vi "FR Measure.vi"(6 "AC sync source":T1, 8 "FR measurement":T6={"Measurement frequencies (Hz)"=[1000.0, 10000.0, 1000.0], "Sampling frequency (Hz)"=500000.0, "Signal amplitude (V)"=4.5, "AC-DC settle time (s)"=20.0, "Record length (multiples of period)"=[1000.0, 10000.0, 1000.0], "Measurement template file"=path "", "Row of START keyword"=0, "Row of STOP keyword"=0, "Calculate RMS from samples"=FALSE, "AC-DC warm up time (s)"=300.0, "Measurement template line"=[], "DC meter readings No."=10, "Algorithm"="TWM-WFFT", "Simultaneous measurement"=FALSE, "Recalculate-skip already calculated"=FALSE} {"Record length (multiples of period)" format="%#_3p"; "Sampling frequency (Hz)" format="%#_3p"; "Measurement frequencies (Hz)" format="%#_3p"}, 9 "DC meter":T4={"DC meter type"=enum."H/A/K 3458", "DC meter VISA"="", "NPLC"=10.0, "status ref"=refnum}, 10 "AC Source":T1, 11 "Common properties":T3={"Measurement status ref"=refnum, "TWM Status ref"=refnum, "Abort ref"=refnum, "Skip waiting ref"=refnum, "GNU Octave path"=path "C:/Program Files/GNU Octave/Octave-6.2.0/mingw64/bin", "TWM+QWTB path"=path "C:/Users/labina/Desktop/TWM-1.8.7.0-full/octprog", "lvlib path"=path "D:/martin/WAC/WACsw - github/control_software/Filter function meter/external libraries/GOLPI 0.7.3.1 source distribution LV 20.0 32 bit/lv_proc.dll", "TWM pipe"="\\\\.\\pipe\\TWM:server", "PJVS status ref"=refnum, "WAC path"=path ""}) -> (0 "error out":errorcluster)   [LabVIEW 2020]
doc: "Main VI to run digitizer frequency response. Setup devices, run loop for all freuencies, stop devices."
uses:
  Type definitions/FR measuement.ctl
  General DC meter/Type definitions/DC meter.ctl
  General DC meter/Type definitions/DC meter type.ctl
  General AC source/Type definitions/AC Source.ctl
  General AC source/Type definitions/AC Source type.ctl
  Utilities/Type definitions/Common properties.ctl
  <vilib>/Utility/error.llb/DialogType.ctl
  <vilib>/Utility/NIReport.llb/NI_report.lvclass
  external libraries/varilib/varilib.lvlib
  external libraries/TWM-1.8.7.0-client/TWM Client.lvlib
panel:
  out "TWM handle":i32
  out "DC readings of AC-AC sequence":dbl[][](array[numeric])
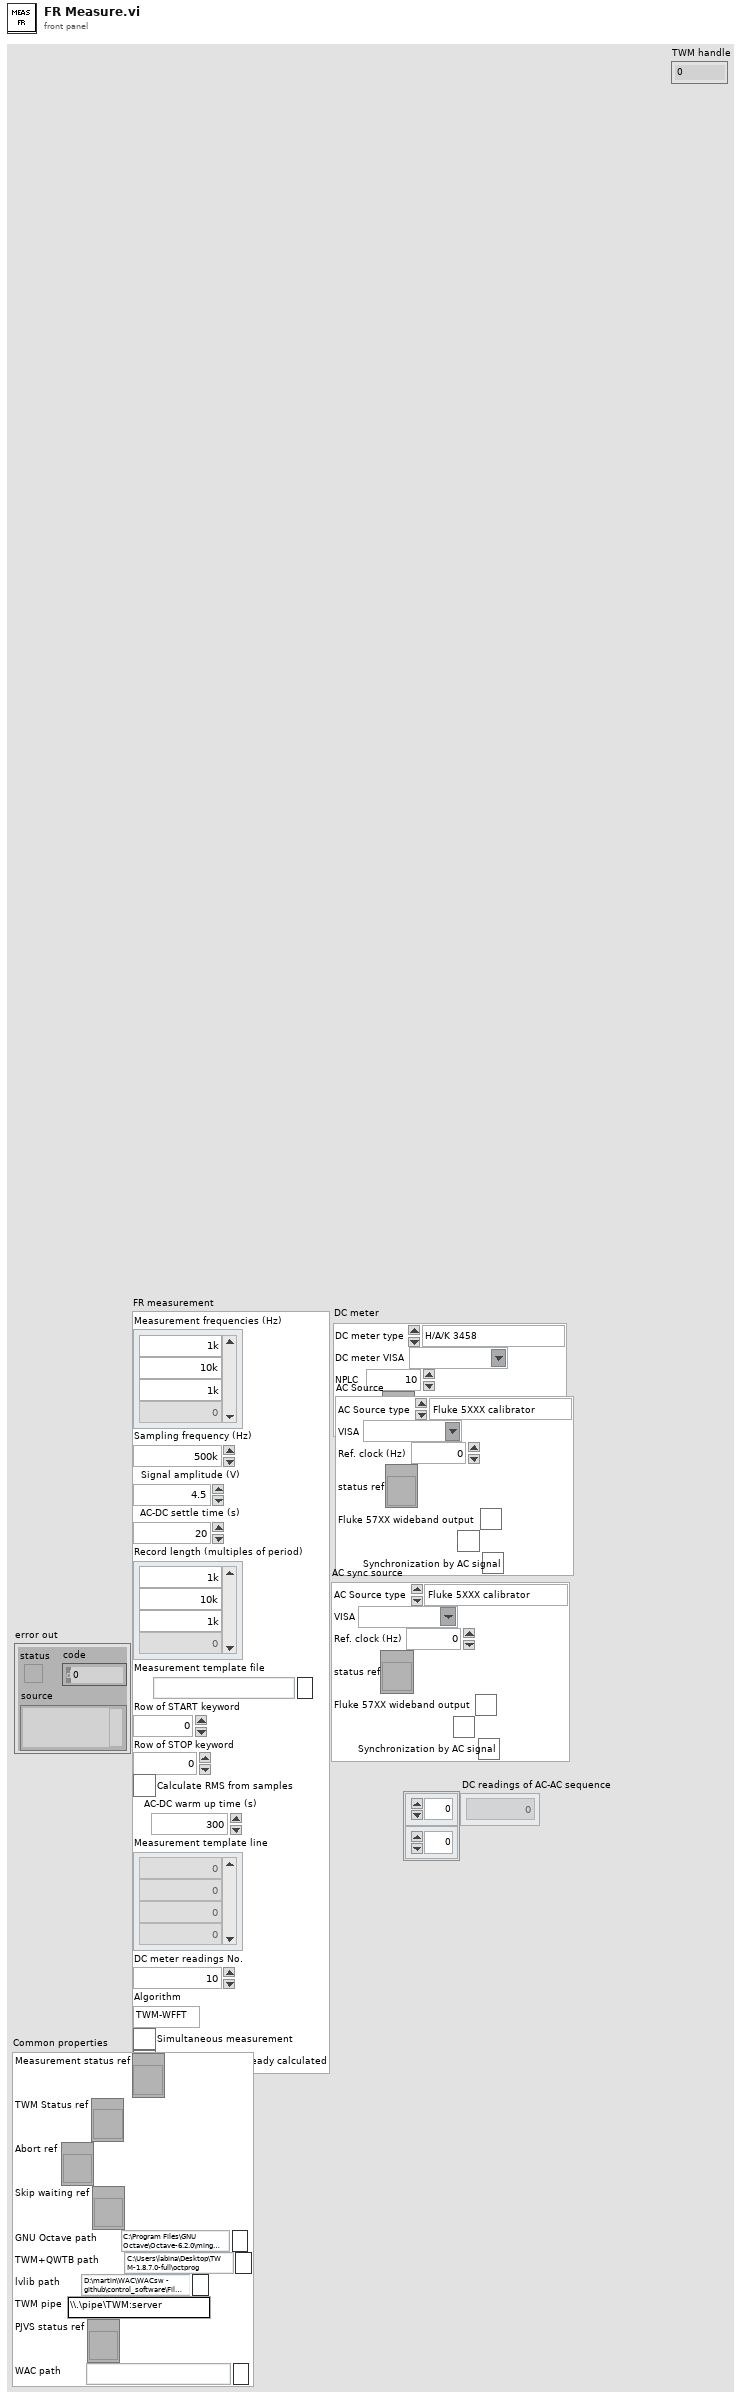
[diagram p1: front panel]
types:
  T1 = typedef "AC Source.ctl" = cluster{"AC Source type":T2, "VISA":refnum<visa-resource-name>, "Ref. clock (Hz)":dbl, "status ref":refnum<vi>, "Fluke 57XX wideband output":bool, "Fluke 57XX ignore errors":bool, "Synchronization by AC signal":bool}
  T2 = typedef "AC Source type.ctl" = enum16{"Fluke 5XXX calibrator", "Tektronix AFG3000 series", "dummy", "Agilent 331xxA to 332xxA", "Agilent 335xxA to 336xxA"}
  T3 = typedef "Common properties.ctl" = cluster{"Measurement status ref":refnum<vi>, "TWM Status ref":refnum<vi>, "Abort ref":refnum<vi>, "Skip waiting ref":refnum<vi>, "GNU Octave path":path, "TWM+QWTB path":path, "lvlib path":path, "TWM pipe":string, "PJVS status ref":refnum<vi>, "WAC path":path}
  T4 = typedef "DC meter.ctl" = cluster{"DC meter type":T5, "DC meter VISA":refnum<visa-resource-name>, "NPLC":dbl, "status ref":refnum<vi>}
  T5 = typedef "DC meter type.ctl" = enum16{"H/A/K 3458", "Fluke 8508A", "dummy", "Keithley 2182"}
  T6 = typedef "FR measuement.ctl" = cluster{"Measurement frequencies (Hz)":dbl[], "Sampling frequency (Hz)":dbl, "Signal amplitude (V)":dbl, "AC-DC settle time (s)":dbl, "Record length (multiples of period)":dbl[], "Measurement template file":path, "Row of START keyword":i32, "Row of STOP keyword":i32, "Calculate RMS from samples":bool, "AC-DC warm up time (s)":dbl, "Measurement template line":i32[], "DC meter readings No.":i32, "Algorithm":string, "Simultaneous measurement":bool, "Recalculate-skip already calculated":bool}
  T7 = typedef "DialogType.ctl" = u16
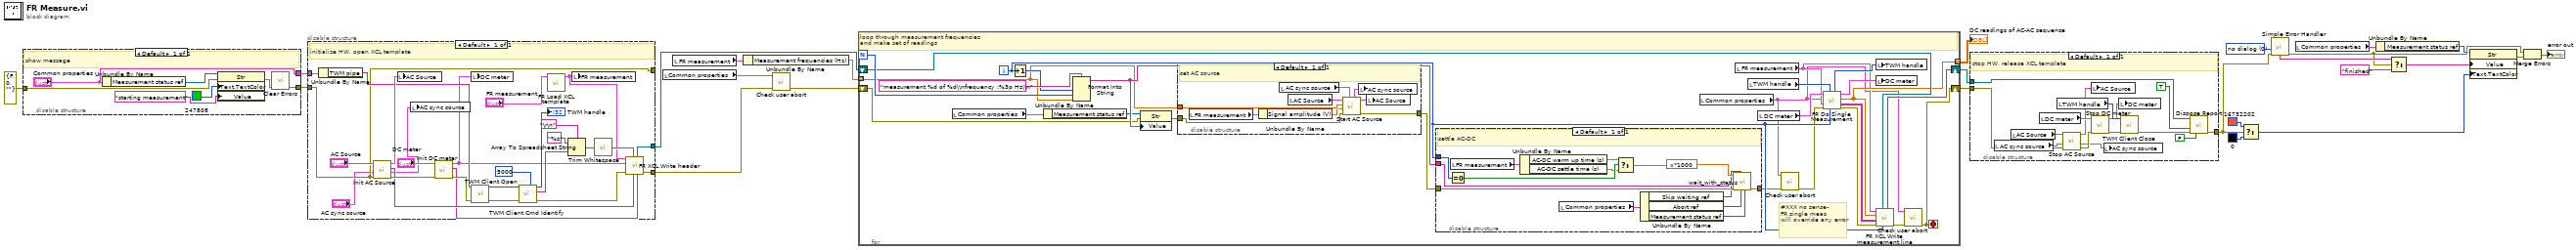
[diagram p0: block diagram]
diagram:
  w21 = T7 0 items=["no dialog", "OK message", "continue or stop message", "OK message + warnings", "continue/stop + warnings"] ("type of dialog (OK msg:1)")
  n1 = disable-structure shown="Default" {
    disable-tunnel: errorcluster {"status"=FALSE, "code"=0, "source"=""} ("error out") -> [w30]
    disable-tunnel: ["Common properties"] -> w2
    disable-tunnel: [w26] -> w1
    frame Enabled {
      # "show message"
      n2 = Unbundle By Name("Common properties") -> ("Measurement status ref"=w27:refnum<vi>)
      n3 = property class="Str"(reference=w27, error in=w30, "Text.TextColor"=u32 247808 ("Text.Text Colors:Text Color"), "Value"="starting measurement") -> (error out=w31:errorcluster)  [unwired: 1 out]
      n4 = call <vilib>:"Clear Errors.vi"("error in (no error)"=w31) -> ("error out"=w26:errorcluster)  [unwired: 5 in, 1 out]
    }
  }
  n5 = disable-structure shown="Default" {
    disable-tunnel: [w35] -> _
    disable-tunnel: [w57] -> w5
    disable-tunnel: [w56] -> w11
    disable-tunnel: w2 -> [w36]
    disable-tunnel: w1 -> [w35]
    frame Enabled {
      # "initialize HW, open XCL template"
      n6 = Unbundle By Name(w36) -> ("TWM pipe"=w40:string)
      n7 = call "Init AC Source.vi"("error in (no error)"=w35, "AC sync source"="AC sync source", "AC source"="AC Source") -> ("error out"=w59:errorcluster, "AC sync source out"=w33:T1, "Init status"=w55:string, "AC source out"=w42:T1)  [unwired: 5 in]
      n8 = local write "AC Source"(w42) -> ()
      n9 = local write "AC sync source"(w33) -> ()
      n10 = call "Init DC meter.vi"("error in (no error)"=w59, "DC meter"="DC meter") -> ("error out"=w58:errorcluster, "Init status"=w54:string, "DC meter out"=w39:T4)  [unwired: 7 in]
      n11 = local write "DC meter"(w39) -> ()
      n12 = call "TWM Client Open.vi"("error in"=w58, "pipe name"=w40) -> ("error out"=w49:errorcluster, "handle out"=w50:i32)  [unwired: 8 in]
      n13 = call "TWM Client Cmd Identify.vi"("timeout [ms]"=5000, "error in"=w49, "handle"=w50) -> ("error out"=w48:errorcluster, "channel idns"=w53:string[], "handle out"=→"TWM handle":i32)  [unwired: 5 in, 1 out]
      n14 = call "FR Load XCL template.vi"("FR measurement"="FR measurement") -> ("FR measurement out"=w37:T6)  [unwired: 10 in]
      n15 = Array To Spreadsheet String(delimiter (Tab)="\r\n", array=w53, 3:"%s" ("format string")) -> (spreadsheet string=w46:string)
      n16 = local write "FR measurement"(w37) -> ()
      n17 = call <vilib>:"Trim Whitespace.vi"("string"=w46) -> ("trimmed string"=w45:string)  [unwired: 1 in]
      n18 = call "FR XCL Write header.vi"("DC meter idn"=w54, "AC source idn"=w55, "Digitizer idn"=w45, "error in (no error)"=w48, "DC meter"=w39, "FR measurement"=w37) -> ("error out"=w57:errorcluster, "NI_report out"=w56:refnum<class "NI_report.lvclass">)  [unwired: 4 in]
    }
  }
  n19 = local read "Common properties"() -> (w3:T3)
  n20 = local read "FR measurement"() -> (w8:T6)
  n21 = Unbundle By Name(w8) -> ("Measurement frequencies (Hz)"=w7:dbl[])
  n22 = call "Check user abort.vi"("error in (no error)"=w5, "Common properties"=w3) -> ("error out"=w4:errorcluster)  [unwired: 9 in]
  n23 = for {
    N -> [w82]
    shift-right: [w66] -> w13
    shift-left: w4 -> [w78]
    tunnel: w7 -> [w79] mode=indexing
    tunnel: [w74] -> w25 mode=indexing
    shift-right: [w76] -> w10
    shift-left: w11 -> [w75]
    i -> [w73]
    stop <- w66 stop-if-true
    # "#XXX no sense-\nFR single meas \nwill override any error"
    # "loop through measurement frequencies\nand make set of readings"
    n24 = local read "Common properties"() -> (w71:T3)
    n25 = Increment(x=w73) -> (x+1=w83:i32)
    n26 = Unbundle By Name(w71) -> ("Measurement status ref"=w70:refnum<vi>)
    n27 = Format Into String(format string="measurement %d of %d\\nfrequency :%3p Hz\\n", w83, w82, w79) -> (resulting string=w84:string)  [unwired: 2 in, 1 out]
    n28 = property class="Str"(reference=w70, error in=w78, "Value"=w84) -> (error out=w81:errorcluster)  [unwired: 1 out]
    n29 = disable-structure shown="Default" {
      disable-tunnel: w81 -> [w108]
      disable-tunnel: [w107] -> w80
      disable-tunnel: w79 -> [w106]
      frame Enabled {
        # "set AC source"
        n30 = local read "FR measurement"() -> (w105:T6)
        n31 = Unbundle By Name(w105) -> ("Signal amplitude (V)"=w104:dbl)
        n32 = local read "AC sync source"() -> (w101:T1)
        n33 = local read "AC Source"() -> (w103:T1)
        n34 = call "Start AC Source.vi"("AC sync source"=w101, "error in (no error)"=w108, "Signal amplitude (V)"=w104, "Signal frequency  (Hz)"=w106, "AC source"=w103) -> ("error out"=w107:errorcluster, "AC source out"=w102:T1, "AC sync source out"=w100:T1)  [unwired: 3 in, 1 out]
        n35 = local write "AC sync source"(w100) -> ()
        n36 = local write "AC Source"(w102) -> ()
      }
    }
    n37 = disable-structure shown="Default" {
      disable-tunnel: w84 -> [w99]
      disable-tunnel: [w96] -> w62
      disable-tunnel: w80 -> [w98]
      disable-tunnel: w73 -> [w95]
      frame Enabled {
        # "settle AC-DC"
        n38 = Equal To 0?(x=w95) -> (x = 0?=w94:bool)
        n39 = local read "FR measurement"() -> (w88:T6)
        n40 = Unbundle By Name(w88) -> ("AC-DC warm up time (s)"=w87:dbl, "AC-DC settle time (s)"=w86:dbl)
        n41 = local read "Common properties"() -> (w92:T3)
        n42 = Select(t=w87, s=w94, f=w86) -> (s? t:f=w93:dbl)
        n43 = Unbundle By Name(w92) -> ("Skip waiting ref"=w91:refnum<vi>, "Abort ref"=w90:refnum<vi>, "Measurement status ref"=w89:refnum<vi>)
        n44 = expression code="x*1000"(w93) -> (w97:dbl)
        n45 = call "wait_with_status.vi"("stat ref"=w89, "stop ref"=w90, "second stop ref"=w91, "error in"=w98, "comment"=w99, "ms to wait"=w97) -> ("error out"=w96:errorcluster)  [unwired: 4 in, 1 out]
      }
    }
    n46 = local read "Common properties"() -> (w60:T3)
    n47 = local read "FR measurement"() -> (w63:T6)
    n48 = local read "TWM handle"() -> (w69:i32)
    n49 = local read "DC meter"() -> (w65:T4)
    n50 = call "Check user abort.vi"("error in (no error)"=w62, "Common properties"=w60) -> ("error out"=w61:errorcluster)  [unwired: 9 in]
    n51 = call "FR Do Single Measurement.vi"("Iteration index"=w73, "TWM handle in"=w69, "error in (no error)"=w61, "FR measurement"=w63, "Common properties"=w60, "DC meter"=w65) -> ("error out"=w77:errorcluster, "TWM result as string"=w72:string[][], "DC readings"=w74:dbl[], "DC meter out"=w64:T4, "TWM handle out"=w68:i32)  [unwired: 1 in]
    n52 = local write "TWM handle"(w68) -> ()
    n53 = local write "DC meter"(w64) -> ()
    n54 = call "FR XCL Write measurement line.vi"("Iteration index"=w73, "report in"=w75, "error in (no error)"=w77, "TWM result as string for XCL"=w72, "DC readings"=w74, "FR measurement"=w63) -> ("error out"=w67:errorcluster, "report out"=w76:refnum<class "NI_report.lvclass">)  [unwired: 4 in]
    n55 = call "Check user abort.vi"("error in (no error)"=w67, "Common properties"=w60) -> ("error out"=w66:errorcluster)  [unwired: 9 in]
  }
  "DC readings of AC-AC sequence" <- w25
  n56 = disable-structure shown="Default" {
    disable-tunnel: [w119] -> w12
    disable-tunnel: w13 -> [w122]
    disable-tunnel: w10 -> [w118]
    frame Enabled {
      # "stop HW, release XCL template"
      n57 = local read "AC sync source"() -> (w110:T1)
      n58 = local read "AC Source"() -> (w112:T1)
      n59 = local read "DC meter"() -> (w114:T4)
      n60 = local read "TWM handle"() -> (w115:i32)
      n61 = call "Stop AC Source.vi"("error in (no error)"=w122, "AC sync source"=w110, "AC source"=w112) -> ("error out"=w123:errorcluster, "AC sync source out"=w109:T1, "AC source out"=w111:T1)  [unwired: 6 in]
      n62 = local write "AC Source"(w111) -> ()
      n63 = call "Stop DC meter.vi"("error in (no error)"=w123, "DC meter"=w114) -> ("error out"=w121:errorcluster, "DC meter out"=w113:T4)  [unwired: 8 in]
      n64 = local write "AC sync source"(w109) -> ()
      n65 = local write "DC meter"(w113) -> ()
      n66 = call "TWM Client Close.vi"("error in"=w121, "handle in"=w115) -> ("error out"=w120:errorcluster)  [unwired: 9 in]
      n67 = call-dynamic "Dispose Report.vi"("report in"=w118, "save changes? (F)"=TRUE, "error in (no error)"=w120, "close report? (T)"=FALSE) -> ("error out"=w119:errorcluster)  [unwired: 11 in]
    }
  }
  n68 = Select(t=u32 16732202 ("Text.Text Colors:Text Color"), s=w12, f=u32 0 ("Text.Text Colors:Text Color")) -> (s? t:f=w18:u32)
  n69 = call <vilib>:"Simple Error Handler.vi"("type of dialog (OK msg:1)"=w21, "error in (no error)"=w12) -> ("error out"=w16:errorcluster, "message"=w24:string)  [unwired: 3 in, 3 out]
  n70 = local read "Common properties"() -> (w6:T3)
  n71 = Unbundle By Name(w6) -> ("Measurement status ref"=w14:refnum<vi>)
  n72 = Select(t=w24, s=w16, f="finished") -> (s? t:f=w22:string)
  n73 = property class="Str"(reference=w14, "Value"=w22, "Text.TextColor"=w18) -> (error out=w17:errorcluster)  [unwired: 1 in, 1 out]
  n74 = Merge Errors(w16, w17) -> (→"error out":errorcluster)
